vi "SVT Pink Noise Waveform.vi"(6 "sampling info":cluster{"Fs":dbl, "#s":dbl}={"Fs"=51200.0, "#s"=1024.0} {"#s" format="%.2f"; "Fs" format="%.2p"}, 7 "reset signal (F)":bool, 8 "error in (no error)":errorcluster, 9 "seed":i32=-1, 11 "amplitude":dbl=1.0 format="%.2f") -> (0 "error out":errorcluster, 3 "pink noise signal":waveform(dbl))   [LabVIEW 2017, in "SoundVib_Generation.lvlib"]
uses:
  <vilib>/addons/_NISVFA/_Generation/SoundVib_Generation.lvlib
  <vilib>/measure/macond.llb/IIR Filter for 1 Chan.vi
  <vilib>/measure/NI_MABase.lvlib
  <vilib>/measure/NI_MAPro.lvlib
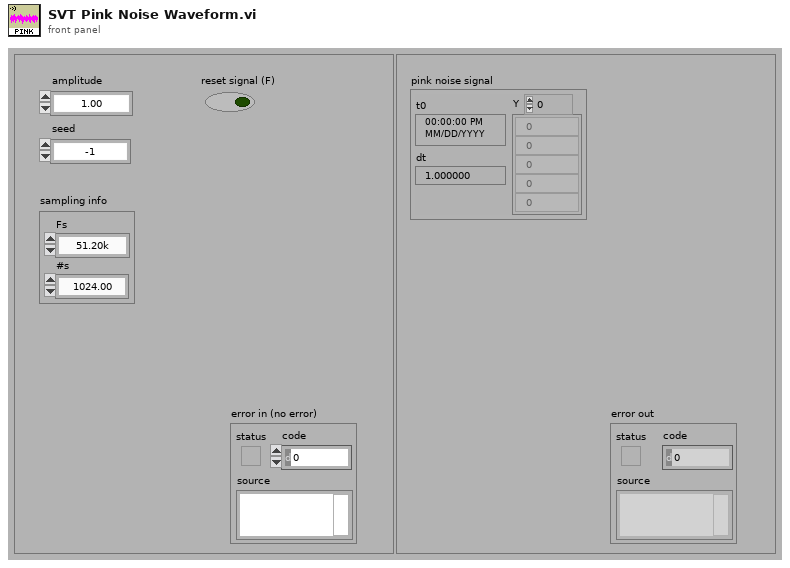
[diagram p1: front panel]
types:
  T1 = cluster{"lower cutoff freq":dbl, "higher cutoff freq":dbl, "order":i32}
  T2 = cluster{"Topology":enum16{"Off", "Butterworth", "Chebyshev", "Inverse Chebyshev", "Elliptic", "Bessel"}, "Type":enum16{"Lowpass", "Highpass", "Bandpass", "Bandstop"}, "Order":i32, "Lower Fc":dbl, "Upper Fc":dbl, "PB Ripple":dbl, "SB Attenuation":dbl}
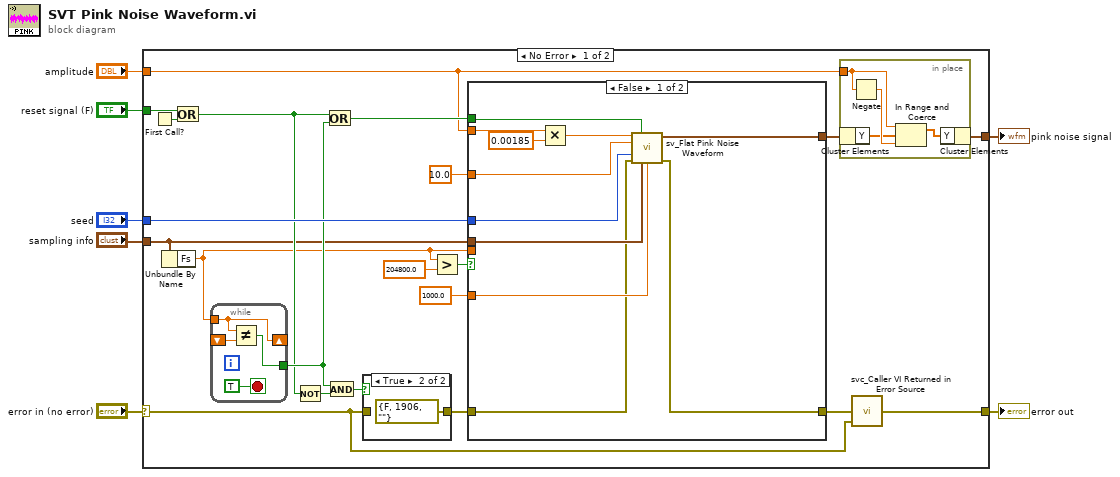
[diagram p0: block diagram]
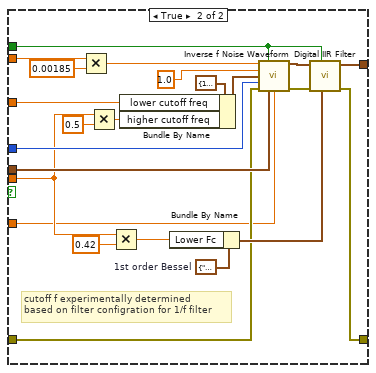
[diagram p2: hidden frame]
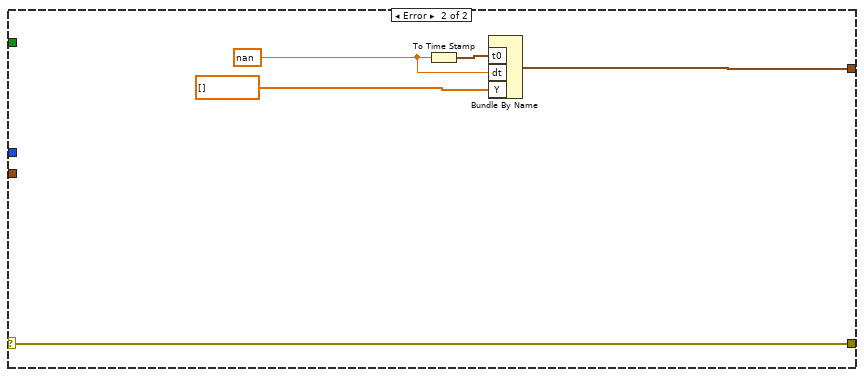
[diagram p4: hidden frame]
diagram:
  n1 = case shown="No Error" "error in (no error)" {
    selector: "error in (no error)" -> [w23 w77]
    tunnel: [w28 w77] -> w6
    tunnel: "sampling info" -> [w11 _]
    tunnel: [w19 w76] -> w5
    tunnel: "amplitude" -> [w8 _]
    tunnel: "seed" -> [w27 _]
    tunnel: "reset signal (F)" -> [w16 _]
    frame No Error {
      n2 = First Call?() -> (First Call?: T/F=w18:bool)
      n3 = Unbundle By Name(w11) -> ("Fs"=w10:dbl)
      n4 = Or(x=w16, y=w18) -> (x .or. y?=w17:bool)
      n5 = while {
        tunnel: [w67] -> w21
        tunnel: w10 -> [w69]
        shift-left: _ -> [w68]
        shift-right: [w69] -> _
        stop <- TRUE stop-if-true
        n6 = Not Equal?(x=w69, y=w68) -> (x != y?=w67:bool)
      }
      n7 = Not(x=w17) -> (.not. x?=w24:bool)
      n8 = Or(x=w17, y=w21) -> (x .or. y?=w20:bool)
      n9 = And(x=w21, y=w24) -> (x .and. y?=w25:bool)
      n10 = case shown="True" w25 {
        tunnel: w23 -> [w71 _]
        tunnel: [w71 errorcluster {"status"=FALSE, "code"=1906, "source"=""} ("error IO")] -> w26
        frame False {
        }
        frame True {
        }
      }
      n11 = Greater?(x=w10, y=204800.0 ("reference freq (Hz)")) -> (0:w14:bool)
      n12 = case shown="False" w14 {
        tunnel: w27 -> [w38 w62]
        tunnel: w26 -> [w33 w45]
        tunnel: w11 -> [w37 w56]
        tunnel: [w32 w49] -> w22
        tunnel: w20 -> [w35 w48]
        tunnel: [w34 w47] -> w9
        tunnel: w10 -> [_ w46]
        tunnel: 1000.0 ("reference freq (Hz)") -> [w36 w44]
        tunnel: 10.0 ("lower cutoff freq") -> [w39 w43]
        tunnel: w8 -> [w30 w41]
        frame False {
          n13 = Multiply(x=w30, y=0.00185 ("ratio of level to amplitude")) -> (x*y=w29:dbl)
          n14 = call <vilib>:"sv_Flat Pink Noise Waveform.vi"("noise density"=w29, "reset signal (F)"=w35, "lower cutoff freq"=w39, "seed"=w38, "error in (no error)"=w33, "sampling info"=w37, "reference freq (Hz)"=w36) -> ("signal out"=w34:waveform(dbl), "error out"=w32:errorcluster)  [unwired: 4 in, 3 out]
        }
        frame True {
          w54 = T2 {"Topology"=enum."Bessel", "Type"=enum."Lowpass", "Order"=1, "Lower Fc"=100.0, "Upper Fc"=200.0, "PB Ripple"=1.0, "SB Attenuation"=60.0}  # 1st order Bessel
          # "cutoff f experimentally determined \nbased on filter configration for 1/f filter"
          n15 = Multiply(x=w41, y=0.00185 ("ratio of level to amplitude")) -> (x*y=w40:dbl)
          n16 = Multiply(x=w46, y=0.5) -> (x*y=w58:dbl)
          n17 = Multiply(x=w46, y=0.42 ("x")) -> (x*y=w55:dbl)
          n18 = Bundle By Name(cluster=T1 {"lower cutoff freq"=10.0, "higher cutoff freq"=100.0, "order"=7} ("filter specifications"), "lower cutoff freq"=w43, "higher cutoff freq"=w58) -> (w57:T1)
          n19 = Bundle By Name(cluster=w54, "Lower Fc"=w55) -> (w50:T2)
          n20 = call <vilib>:"Inverse f Noise Waveform.vi"("noise density"=w40, "reset signal (F)"=w48, "exponent"=1.0, "filter specifications"=w57, "seed"=w62, "error in (no error)"=w45, "sampling info"=w56, "reference freq (Hz)"=w44) -> ("signal out"=w52:waveform(dbl), "error out"=w51:errorcluster)  [unwired: 3 in, 3 out]
          n21 = call-poly <vilib>:"Digital IIR Filter.vi"("IIR filter specifications"=w50, "reset filter"=w48, "error in (no error)"=w51, "signal in"=w52) -> ("error out"=w49:errorcluster, "signal out"=w47:waveform(dbl))  [unwired: 5 in, 1 out]
        }
      }
      n22 = in-place {
        in-place-border: w8 -> [w65]
        n23 = in-place-cluster #1(w9) -> ("Y"=w64:dbl[])
        n24 = Negate(x=w65) -> (-x=w66:dbl)
        n25 = In Range and Coerce(upper limit=w65, x=w64, lower limit=w66) -> (coerced(x)=w63:dbl[])  [unwired: 1 out]
        n26 = in-place-cluster #1("Y"=w63) -> (w19:waveform(dbl))
      }
      n27 = call <vilib>:"svc_Caller VI Returned in Error Source.vi"("warning input to caller"=w23, "error in (no error)"=w22) -> ("error out"=w28:errorcluster)  [unwired: 3 in]
    }
    frame Error {
      w73 = nan ("t0")
      n28 = To Time Stamp(1:w73) -> (0:w74:timestamp)
      n29 = Bundle By Name("t0"=w74, "dt"=w73, "Y"=dbl[] []) -> (w76:waveform(dbl))  [unwired: 1 in]
    }
  }
  "error out" <- w6
  "pink noise signal" <- w5
